vi "Update.vi"(8 "error in (no error)":errorcluster, 11 "FadeOutTiles in":refnum<class "FadeOutTiles.lvclass">) -> (0 "error out":errorcluster, 2 "Done?":bool, 3 "FadeOutTiles out":refnum<class "FadeOutTiles.lvclass">)   [LabVIEW 2019, in "RT_Game.lvlib" / "FadeOutTiles.lvclass"]
uses:
  FadeOutTiles.lvclass
  FadeOutTiles.lvclass/FadeOutTiles.ctl
  Engine/Globals.vi
  Engine/Engine.lvclass
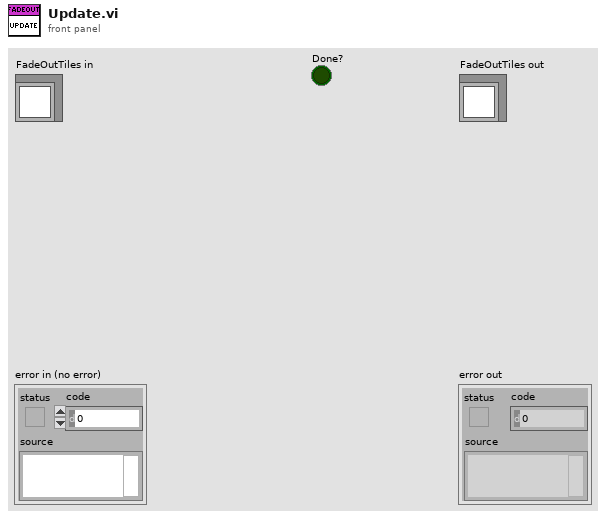
[diagram p1: front panel]
types:
  T1 = typedef "RT_Game.lvlib/Engine.lvclass/TileCoordinate.ctl" = cluster{"x":i16, "y":i16}
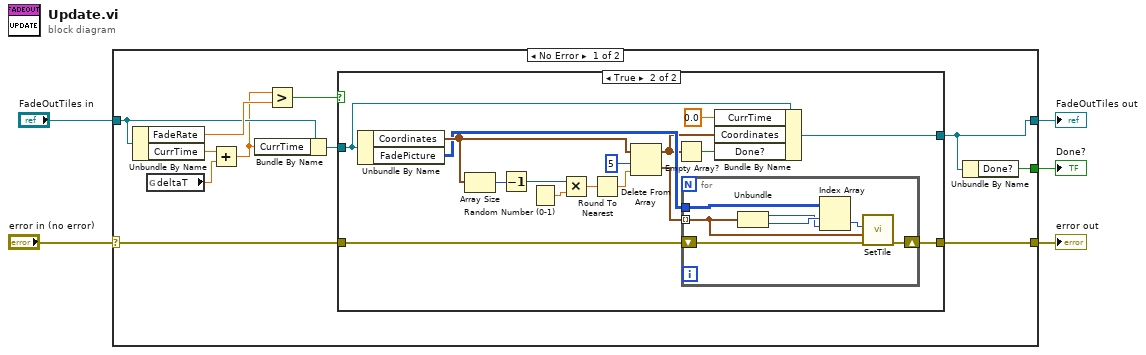
[diagram p0: block diagram]
diagram:
  n1 = case shown="No Error" "error in (no error)" {
    selector: "error in (no error)" -> [w16 w43]
    tunnel: [w12 w43] -> w4
    tunnel: [w6 w42] -> w2
    tunnel: "FadeOutTiles in" -> [w9 w42]
    tunnel: [w15 _] -> w1
    frame No Error {
      n2 = Unbundle By Name(w9) -> ("FadeRate"=w10:dbl, "CurrTime"=w14:dbl)
      n3 = global read "Globals.vi" "deltaT"() -> (w13:dbl)
      n4 = Add(x=w14, y=w13) -> (x+y=w7:dbl)
      n5 = Bundle By Name(cluster=w9, "CurrTime"=w7) -> (w8:refnum<class "FadeOutTiles.lvclass">)
      n6 = Greater?(x=w7, y=w10) -> (0:w11:bool)
      n7 = case shown="True" w11 {
        tunnel: w16 -> [w18 w34]
        tunnel: [w18 w33] -> w12
        tunnel: w8 -> [w17 w26]
        tunnel: [w17 w25] -> w6
        frame False {
        }
        frame True {
          n8 = Unbundle By Name(w26) -> ("Coordinates"=w27:T1[], "FadePicture"=w22:u32[][])
          n9 = Array Size(array=w27) -> (size(s)=w32:i32)
          n10 = Decrement(x=w32) -> (x-1=w28:i32)
          n11 = Random Number (0-1)() -> (number: 0 to 1=w31:dbl)
          n12 = Multiply(x=w28, y=w31) -> (x*y=w30:dbl)
          n13 = Round To Nearest(number=w30) -> (nearest integer value=w29:dbl)
          n14 = Delete From Array(array=w27, length=5, index=w29) -> (deleted portion=w23:T1[], array with subset deleted=w21:T1[])
          n15 = Empty Array?(array=w21) -> (empty?=w20:bool)
          n16 = for {
            tunnel: w23 -> [w39] mode=indexing
            tunnel: w22 -> [w37]
            shift-right: [w40] -> w33
            shift-left: w34 -> [w41]
            n17 = Unbundle(w39) -> ("x"=w36:i16, "y"=w38:i16)
            n18 = Index Array(array=w37, index (row)=w38, index (col)=w36) -> (element=w35:u32)
            n19 = call "SetTile.vi"("error in (no error)"=w41, "Coordinates"=w39, "TileCode"=w35) -> ("error out"=w40:errorcluster)  [unwired: 8 in]
          }
          n20 = Bundle By Name(cluster=w26, "CurrTime"=0.0, "Coordinates"=w21, "Done?"=w20) -> (w25:refnum<class "FadeOutTiles.lvclass">)
        }
      }
      n21 = Unbundle By Name(w6) -> ("Done?"=w15:bool)
    }
    frame Error {
    }
  }
  "error out" <- w4
  "FadeOutTiles out" <- w2
  "Done?" <- w1
